vi "Project_labview_1.vi"() -> ()   [LabVIEW 2020]
panel:
  in  "Table Control":string[][](table)
  out "Moisture Sensor":dbl(graph)
  out "Stop Flow Out":bool
  out "Moisture-Level":dbl(knob) scale=0.0..100.0
  out "Water-level Sensor":dbl(graph)
  in  "VISA Resource Port":refnum<visa-resource-name>
  out "TURN PUMP ON":bool
  out "TURN PUMP  OFF":bool
  out "Tank (Liters/sec)":dbl(slide) scale=0.0..100.0
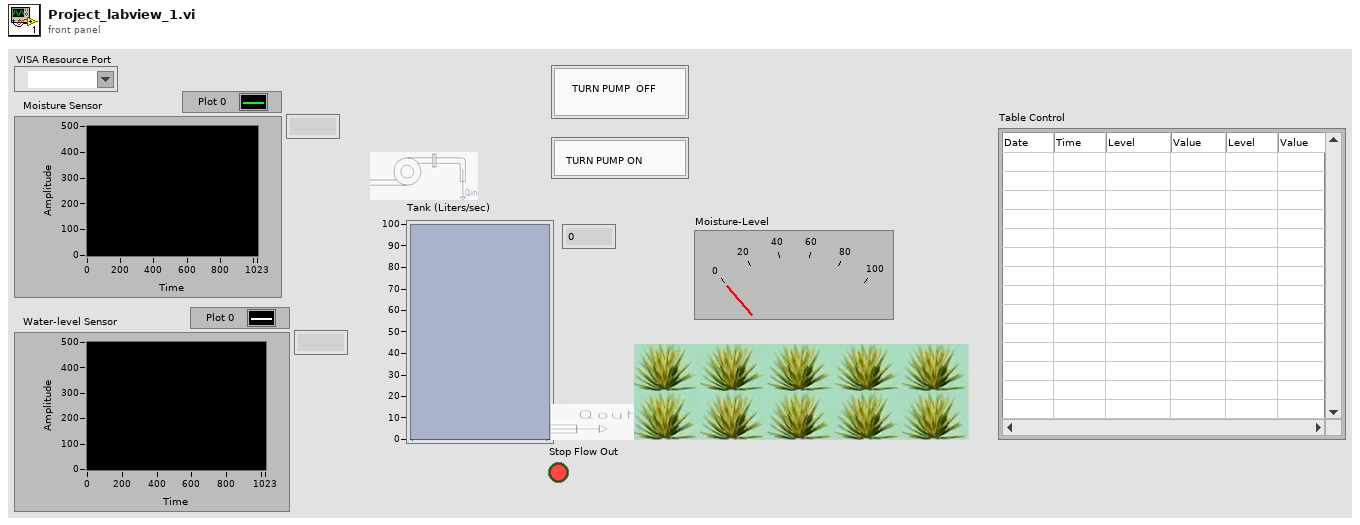
[diagram p1: front panel]
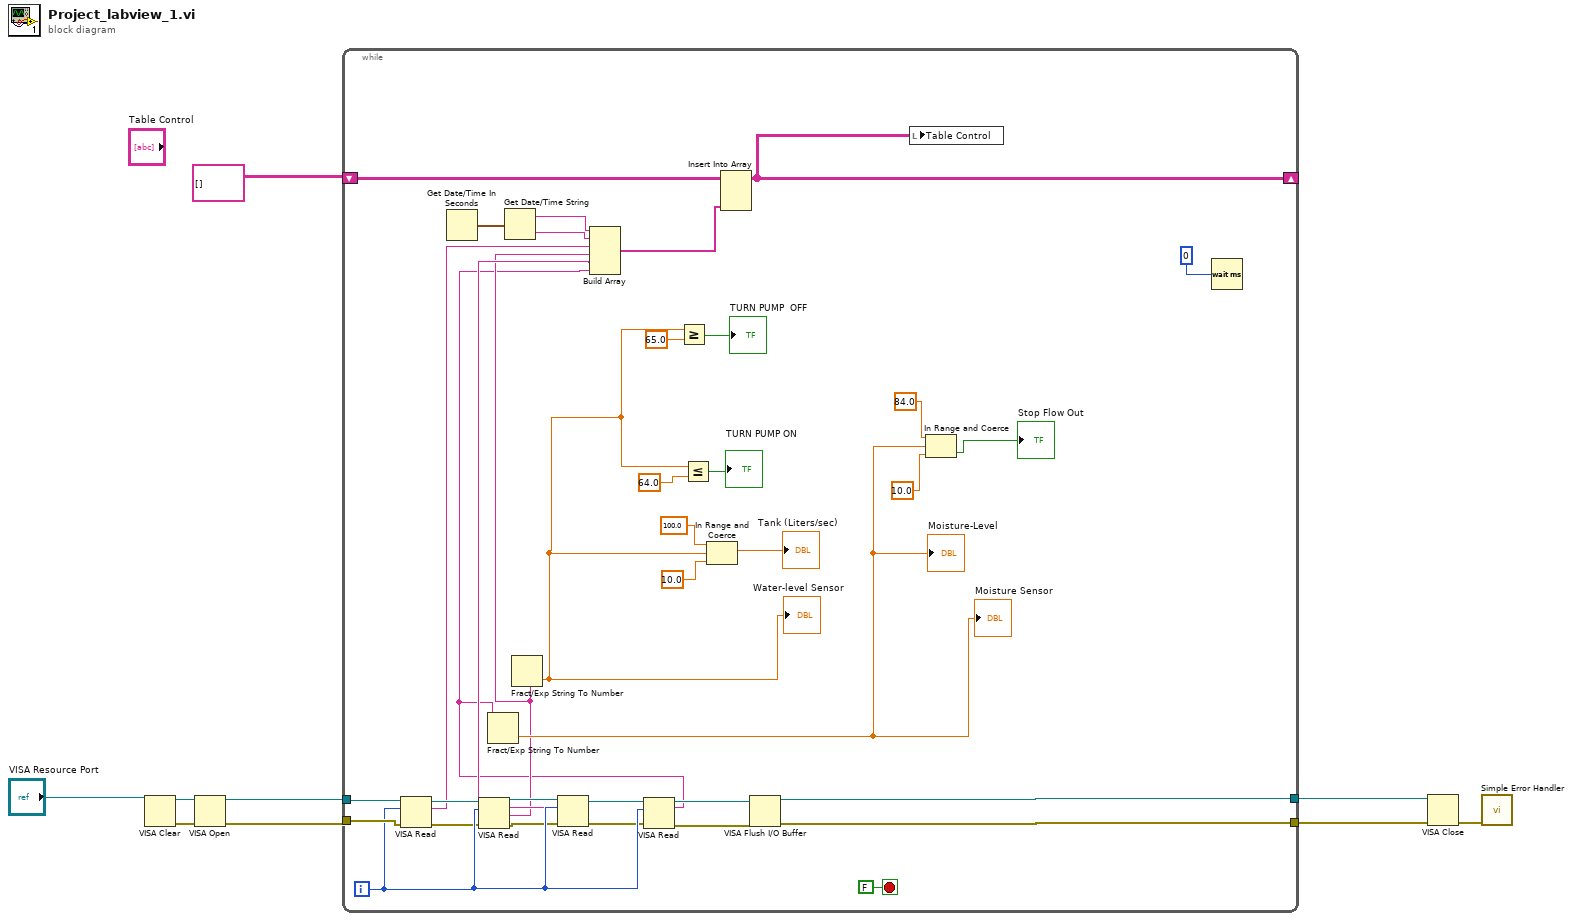
[diagram p0: block diagram]
diagram:
  n1 = VISA Clear(VISA resource name="VISA Resource Port") -> (VISA resource name out=w8:refnum<visa-resource-name>, error out=w9:errorcluster)  [unwired: 1 in]
  n2 = VISA Open(error in (no error)=w9, VISA resource name=w8) -> (VISA resource name=w7:refnum<visa-resource-name>, error out=w6:errorcluster)  [unwired: 3 in]
  n3 = while {
    tunnel: w7 -> [w21]
    tunnel: w6 -> [w20]
    tunnel: [w39] -> w5
    tunnel: [w38] -> w4
    shift-right: [w31] -> _
    shift-left: string[][] [] -> [w32]
    i -> [w19]
    stop <- FALSE stop-if-true
    n4 = VISA Read(VISA resource name=w21, byte count=w19, error in (no error)=w20) -> (VISA resource name out=w22:refnum<visa-resource-name>, read buffer=w13:string, error out=w14:errorcluster)  [unwired: 1 out]
    n5 = Get Date/Time In Seconds() -> (seconds since 1Jan1904=w30:timestamp)
    n6 = VISA Read(VISA resource name=w22, byte count=w19, error in (no error)=w14) -> (VISA resource name out=w18:refnum<visa-resource-name>, read buffer=w11:string, error out=w17:errorcluster)  [unwired: 1 out]
    n7 = Get Date/Time String(seconds (now)=w30) -> (date string=w29:string, time string=w28:string)  [unwired: 2 in]
    n8 = Fract/Exp String To Number(string=w11) -> (number=w26:dbl)  [unwired: 3 in, 1 out]
    "Water-level Sensor" <- w26
    n9 = VISA Read(VISA resource name=w18, byte count=w19, error in (no error)=w17) -> (VISA resource name out=w16:refnum<visa-resource-name>, read buffer=w12:string, error out=w15:errorcluster)  [unwired: 1 out]
    n10 = VISA Read(VISA resource name=w16, byte count=w19, error in (no error)=w15) -> (VISA resource name out=w41:refnum<visa-resource-name>, read buffer=w10:string, error out=w40:errorcluster)  [unwired: 1 out]
    n11 = Fract/Exp String To Number(string=w10) -> (number=w34:dbl)  [unwired: 3 in, 1 out]
    "Moisture-Level" <- w34
    "Moisture Sensor" <- w34
    n12 = Build Array(w29, w28, w13, w11, w12, w10) -> (w27:string[])
    n13 = Greater Or Equal?(x=w26, y=65.0) -> (x >= y?=→"TURN PUMP  OFF":bool)
    n14 = Less Or Equal?(x=w26, y=64.0) -> (x <= y?=→"TURN PUMP ON":bool)
    n15 = In Range and Coerce(upper limit=100.0, x=w26, lower limit=10.0) -> (coerced(x)=→"Tank (Liters/sec)":dbl)  [unwired: 1 out]
    n16 = Insert Into Array(array=w32, new element=w27) -> (w31:string[][])  [unwired: 2 in]
    n17 = VISA Flush I/O Buffer(VISA resource name=w41, error in (no error)=w40) -> (VISA resource name out=w39:refnum<visa-resource-name>, error out=w38:errorcluster)  [unwired: 1 in]
    n18 = local write "Table Control"(w31) -> ()
    n19 = In Range and Coerce(upper limit=84.0, x=w34, lower limit=10.0) -> (In Range?=→"Stop Flow Out":bool)  [unwired: 1 out]
    n20 = Wait (ms)(milliseconds to wait=u32 0) -> ()  [unwired: 1 out]
  }
  n21 = VISA Close(VISA resource name=w5, error in (no error)=w4) -> (error out=w2:errorcluster)
  n22 = call <vilib>:"Simple Error Handler.vi"("error in (no error)"=w2) -> ()  [unwired: 4 in, 5 out]
